vi "ReportError.vi"(8 "error in (no error)":errorcluster, 10 "ErrorReported":errorcluster, 11 "ModuleID":i32) -> (0 "error out":errorcluster)   [LabVIEW 2018, in "SensorPlugins.lvlib"]
uses:
  SensorPlugins/SensorPlugins.lvlib
  SensorShared/clEventType.ctl
  SensorShared/SensorShared.lvlib
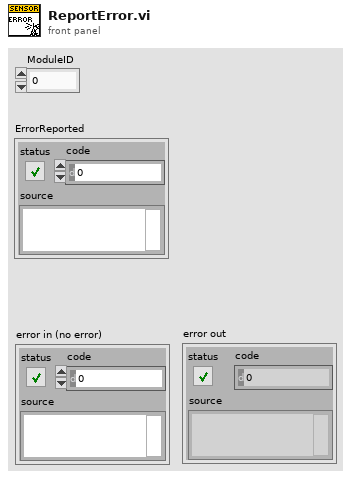
[diagram p1: front panel]
types:
  T1 = typedef "SensorShared.lvlib/clEventType.ctl" = cluster{"ModuleID":i32, "Data":variant}
  T2 = typedef "SensorShared.lvlib/clBroadcastEvents.ctl" = cluster{"DidInit":refnum<user-event>, "StatusUpdate":refnum<user-event>, "ErrorReport":refnum<user-event>, "DidStop":refnum<user-event>, "PathToINI":refnum<user-event>, "SensorReport":refnum<user-event>, "SensorConfig":refnum<user-event>}
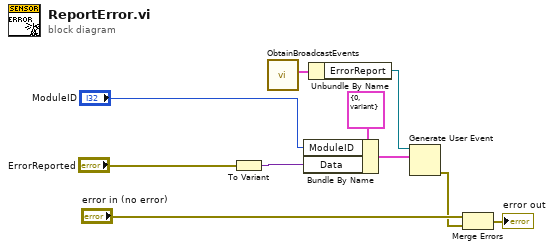
[diagram p0: block diagram]
diagram:
  n1 = To Variant(anything="ErrorReported") -> (Variant=w9:variant)
  n2 = call "ObtainBroadcastEvents.vi"() -> ("clBroadcastEvents"=w7:T2)  [unwired: 10 in, 1 out]
  n3 = Bundle By Name(cluster=T1 {"ModuleID"=0, "Data"=variant} ("clEventType"), "ModuleID"="ModuleID", "Data"=w9) -> (w6:T1)
  n4 = Unbundle By Name(w7) -> ("ErrorReport"=w5:refnum<user-event>)
  n5 = Generate User Event(user event=w5, event data cluster=w6) -> (error out=w2:errorcluster)  [unwired: 2 in, 1 out]
  n6 = Merge Errors("error in (no error)", w2) -> (→"error out":errorcluster)
